vi "ValueSignalLatchBooleanArray.vi"(0 "VI Reference In":refnum<vi>, 5 "Control Path":string[](array[string]), 11 "error in":errorcluster) -> (4 "VI Reference Out":refnum<vi>, 15 "error out":errorcluster)   [LabVIEW 2016, in "Drona.lvlib" / "KeyboardSimulation.lvlib"]
doc: "Triggers the latch boolean by keyboard simulation.\n\nThe path of the control should be given in the successive index of the array"
uses:
  KeyboardSimulation.lvlib
  Get/GetControlRef/GetControlRef.lvlib
  VI/VI.lvlib
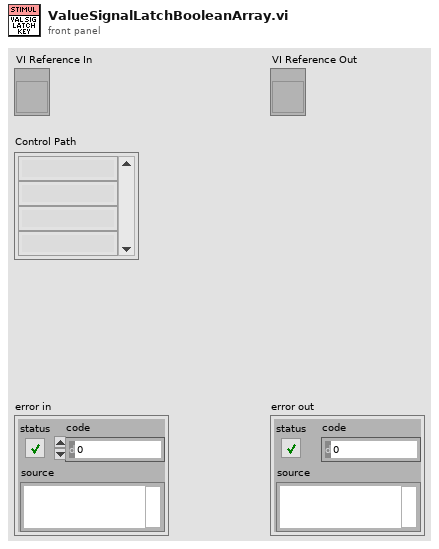
[diagram p1: front panel]
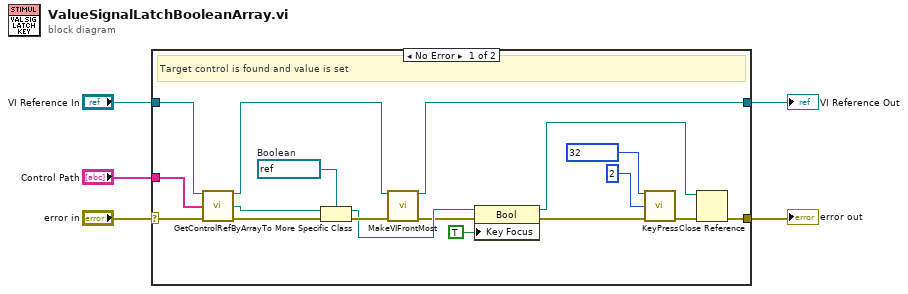
[diagram p0: block diagram]
diagram:
  n1 = case shown="No Error" "error in" {
    selector: "error in" -> [w23 w25]
    tunnel: "Control Path" -> [w20 _]
    tunnel: "VI Reference In" -> [w19 w24]
    tunnel: [w14 w24] -> w2
    tunnel: [w18 w25] -> w1
    frame No Error {
      w12 = refnum<vi> refnum  # Boolean
      # "Target control is found and value is set"
      n2 = call "GetControlRefByArray.vi"("VI Reference In"=w19, "Control Path"=w20, "error In"=w23) -> ("VI Reference Out"=w15:refnum<vi>, "Ctl Refnum"=w16:refnum<vi>, "error out"=w22:errorcluster)  [unwired: 10 in]
      n3 = To More Specific Class(target class=w12, reference=w16, error in=w22) -> (specific class reference=w11:refnum<vi>, error out=w13:errorcluster)
      n4 = call "MakeVIFrontMost.vi"("VI Reference In"=w15, "error in"=w13) -> ("VI Reference Out"=w14:refnum<vi>, "error out"=w10:errorcluster)  [unwired: 12 in]
      n5 = property class="Bool"(reference=w11, error in=w10, "Key Focus"=TRUE) -> (reference out=w17:refnum<vi>, error out=w9:errorcluster)
      n6 = call "KeyPress.vi"("Virtual Key"=u8 32, "Millis"=u32 2, "error in"=w9) -> ("error out"=w21:errorcluster)  [unwired: 12 in]
      n7 = Close Reference(reference=w17, error in (no error)=w21) -> (error out=w18:errorcluster)
    }
    frame Error {
    }
  }
  "error out" <- w1
  "VI Reference Out" <- w2
